vi "Read Measurement (FSK Demodulation).vi"(0 "VISA resource name":refnum<visa-resource-name>, 11 "error in (no error)":errorcluster) -> (3 "Carrier Power (dBm)":dbl[](array[numeric]), 4 "VISA resource name out":refnum<visa-resource-name>, 6 "Deviation (Hz)":dbl[](array[numeric]), 8 "FSK Error (%)":dbl[](array[numeric]), 10 "Mag Error (%)":dbl[](array[numeric]), 14 "Carrier Frequency Offset (Hz)":dbl[](array[numeric]), 15 "error out":errorcluster)   [LabVIEW 2022 SP3, in "Agilent N934X Series.lvlib"]
doc: "Reads the measurement result from the spectrum analyzer (FM Demodulation Measurement).\n\nNotes:\n\n(1) This VI is only available for N9321C, N9322C, N9323C, N9324C models.\n(2) User must use <B>Configure Measurement Type.vi</B> to change the mode to <B>FSK Modulation</B> before using this VI."
uses:
  <instrlib>/Agilent N934X Series/Agilent N934X Series.lvlib
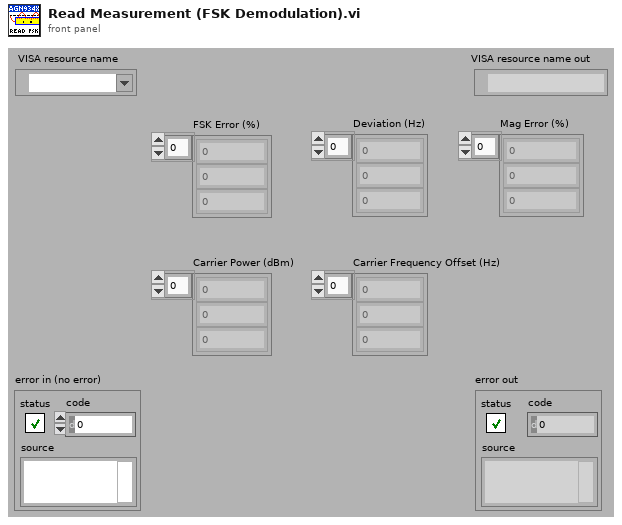
[diagram p1: front panel]
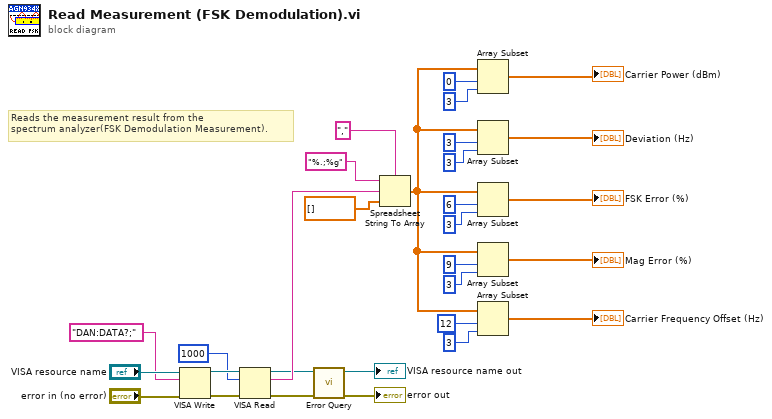
[diagram p0: block diagram]
diagram:
  # "Reads the measurement result from the \nspectrum analyzer(FSK Demodulation Measurement)."
  n1 = VISA Write(VISA resource name="VISA resource name", write buffer="DAN:DATA?;", error in (no error)="error in (no error)") -> (VISA resource name out=w29:refnum<visa-resource-name>, error out=w30:errorcluster)  [unwired: 1 out]
  n2 = VISA Read(VISA resource name=w29, byte count=u32 1000, error in (no error)=w30) -> (VISA resource name out=w1:refnum<visa-resource-name>, read buffer=w21:string, error out=w2:errorcluster)  [unwired: 1 out]
  n3 = call <instrlib>:"Error Query.vi"("error in (no error)"=w2, "VISA resource name"=w1) -> ("error out"=→"error out":errorcluster, "VISA resource name out"=→"VISA resource name out":refnum<visa-resource-name>)  [unwired: 6 in, 2 out]
  n4 = Spreadsheet String To Array(delimiter (Tab)=",", format string="%.;%g", spreadsheet string=w21, array type (2D Dbl)=dbl[] [] ("Measurement Data 2")) -> (array=w10:dbl[])
  n5 = Array Subset(array=w10, index=0, length=3) -> (→"Carrier Power (dBm)":dbl[])
  n6 = Array Subset(array=w10, index=3, length=3) -> (→"Deviation (Hz)":dbl[])
  n7 = Array Subset(array=w10, index=6, length=3) -> (→"FSK Error (%)":dbl[])
  n8 = Array Subset(array=w10, index=9, length=3) -> (→"Mag Error (%)":dbl[])
  n9 = Array Subset(array=w10, index=12, length=3) -> (→"Carrier Frequency Offset (Hz)":dbl[])
